vi "niLvFpga_Open_cRIO-9104.vi"(0 "device name":T2, 1 "what the device is doing":T1=enum."FPGA interface", 2 "signature":u8[](array[numeric]), 5 "bitfileInfo":string, 7 "run when opened":bool, 9 "Force Download (F)":bool, 11 "error in":errorcluster, 12 "vi signatures match":bool, 13 "node name for error reporting":string) -> (4 "session out":u32, 15 "error out":errorcluster)   [LabVIEW 2017]
uses:
  <vilib>/userdefined/High Color/nirio_resource_hc.ctl
  <vilib>/rvi/ClientSDK/nirviWhatTheDeviceIsDoing.ctl
  NiFpgaLv.dll
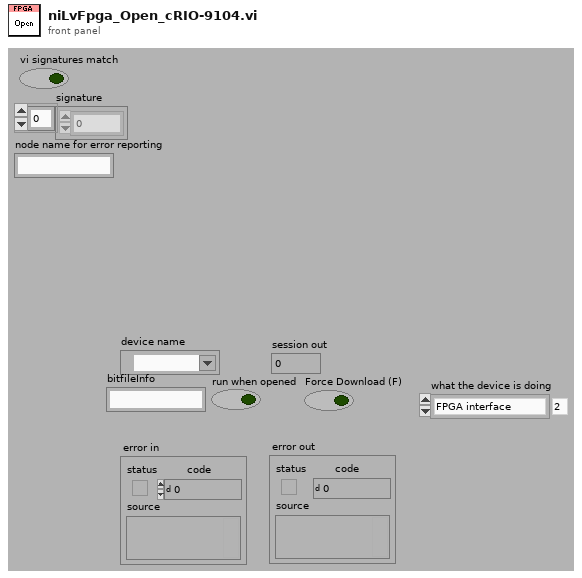
[diagram p1: front panel]
types:
  T1 = typedef "nirviWhatTheDeviceIsDoing.ctl" = enum32{"C Interface", "RIO Scan Interface", "FPGA interface", "Interactive Mode", "Emulation Mode"}
  T2 = typedef "nirio_resource_hc.ctl" = tag
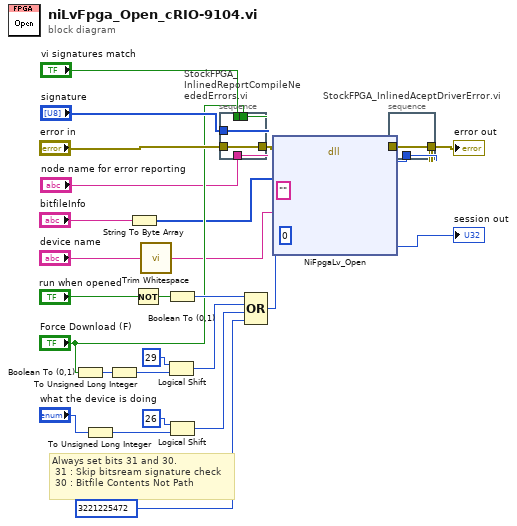
[diagram p0: block diagram]
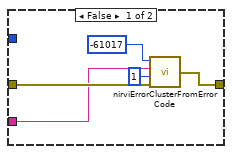
[diagram p3: hidden frame]
diagram:
  # "Always set bits 31 and 30.\n 31 : Skip bitsream signature check\n 30 : Bitfile Contents Not Path"
  n1 = Boolean To (0,1)(Boolean="Force Download (F)") -> (0, 1=w15:i16)
  n2 = To Unsigned Long Integer(number="what the device is doing") -> (unsigned 32bit integer=w19:u32)
  n3 = To Unsigned Long Integer(number=w15) -> (unsigned 32bit integer=w17:u32)
  n4 = String To Byte Array(string="bitfileInfo") -> (unsigned byte array=w3:u8[])
  n5 = Not(x="run when opened") -> (.not. x?=w12:bool)
  n6 = call <vilib>:"Trim Whitespace.vi"("string"="device name") -> ("trimmed string"=w1:string)  [unwired: 1 in]
  n7 = Logical Shift(y=u32 29 ("x"), x=w17) -> (x << y=w14:u32)
  n8 = Boolean To (0,1)(Boolean=w12) -> (0, 1=w11:i16)
  n9 = Logical Shift(y=u32 26 ("x"), x=w19) -> (x << y=w22:u32)
  n10 = stacked-sequence "StockFPGA_InlinedReportCompileNeededErrors.vi" {
    tunnel: "vi signatures match" -> [w33]
    tunnel: "Force Download (F)" -> [w34]
    tunnel: "signature" -> [w32]
    tunnel: "error in" -> [w35]
    tunnel: "node name for error reporting" -> [w31]
    tunnel: [w30] -> w8
    frame #0 {
      n11 = case shown="No Error" w35 {
        selector: w35 -> [w37 w59]
        tunnel: [w43 w59] -> w30
        tunnel: w31 -> [w42 _]
        tunnel: w32 -> [w40 _]
        tunnel: w33 -> [w39 _]
        tunnel: w34 -> [w38 _]
        frame No Error {
          n12 = Array Size(array=w40) -> (size(s)=w36:i32)
          n13 = Or(x=w38, y=w39) -> (x .or. y?=w41:bool)
          n14 = case shown="True" w41 {
            tunnel: w37 -> [w46 w51]
            tunnel: w36 -> [_ w52]
            tunnel: [w47 w49] -> w43
            tunnel: w42 -> [w45 w50]
            frame False {
              n15 = call <vilib>:"nirviErrorClusterFromErrorCode.vi"("error code"=-61017 ("[error code] (0)"), "Function Name"=w45, "levels of hierarchy to ignore"=1, "error in"=w46) -> ("error out"=w47:errorcluster)  [unwired: 1 in]
            }
            frame True {
              n16 = case shown="..0" w52 {
                tunnel: w51 -> [w56 w58]
                tunnel: [w55 w58] -> w49
                tunnel: w50 -> [w54 _]
                frame ..0 {
                  n17 = call <vilib>:"nirviErrorClusterFromErrorCode.vi"("error code"=-61016 ("[error code] (0)"), "Function Name"=w54, "levels of hierarchy to ignore"=1, "error in"=w56) -> ("error out"=w55:errorcluster)  [unwired: 1 in]
                }
                frame 1.. {
                }
              }
            }
          }
        }
        frame Error {
        }
      }
    }
  }
  n18 = Compound Arithmetic op=OR(w11, w14, w22, u32 3221225472 ("x")) -> (w21:u32)
  n19 = dll-call lib="NiFpgaLv.*" fn="NiFpgaLv_Open" label="niLvFpgaOpen"(error in=w8, "bitfileInfo"=w3, "apiSignature"="", "resource"=w1, "attribute"=w21, "session"=u32 0 ("session in")) -> (error out=w28:errorcluster, "status"=w27:i32, "session"=→"session out":u32)  [unwired: 4 in, 3 out]
  n20 = stacked-sequence "StockFPGA_InlinedAceptDriverError.vi" {
    tunnel: w28 -> [w60]
    tunnel: w27 -> [w62]
    tunnel: [w61] -> w26
    frame #0 {
      n21 = case shown="Default" w62 {
        selector: w62 -> [_ w64]
        tunnel: [w63 w66] -> w61
        tunnel: w60 -> [w63 w67]
        frame 0 {
        }
        frame Default {
          n22 = Greater Than 0?(x=w64) -> (x > 0?=w65:bool)
          n23 = call <vilib>:"Error Cluster From Error Code.vi"("is warning? (False)"=w65, "error in (no error)"=w67, "error code (0)"=w64) -> ("error out"=w66:errorcluster)  [unwired: 6 in]
        }
      }
    }
  }
  "error out" <- w26
